vi "GVZwangsMPV.vi"() -> ()   [LabVIEW 2017]
panel:
  out "ZwangsMPV?":bool
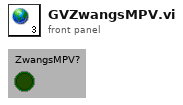
[diagram p1: front panel]
diagram:
